vi "Load DXF 2.vi"(7 "DXF Options":T1={"Pen Up Z"=20.0, "Pen Down Z"=-50.0, "Speed"=1500.0, "Z Move Speed"=300.0}, 8 "error in (no error)":errorcluster, 9 "Trigger (SEQEND)":string="SEQEND", 11 "String in":string) -> (0 "error out":errorcluster, 1 "String Array":string[](array[string]), 3 "Command Array":T2[](array[typedef]))   [LabVIEW 2014]
uses:
  GCode Parser/GCode Command Cluster.ctl
panel:
  out "Numeric":i32
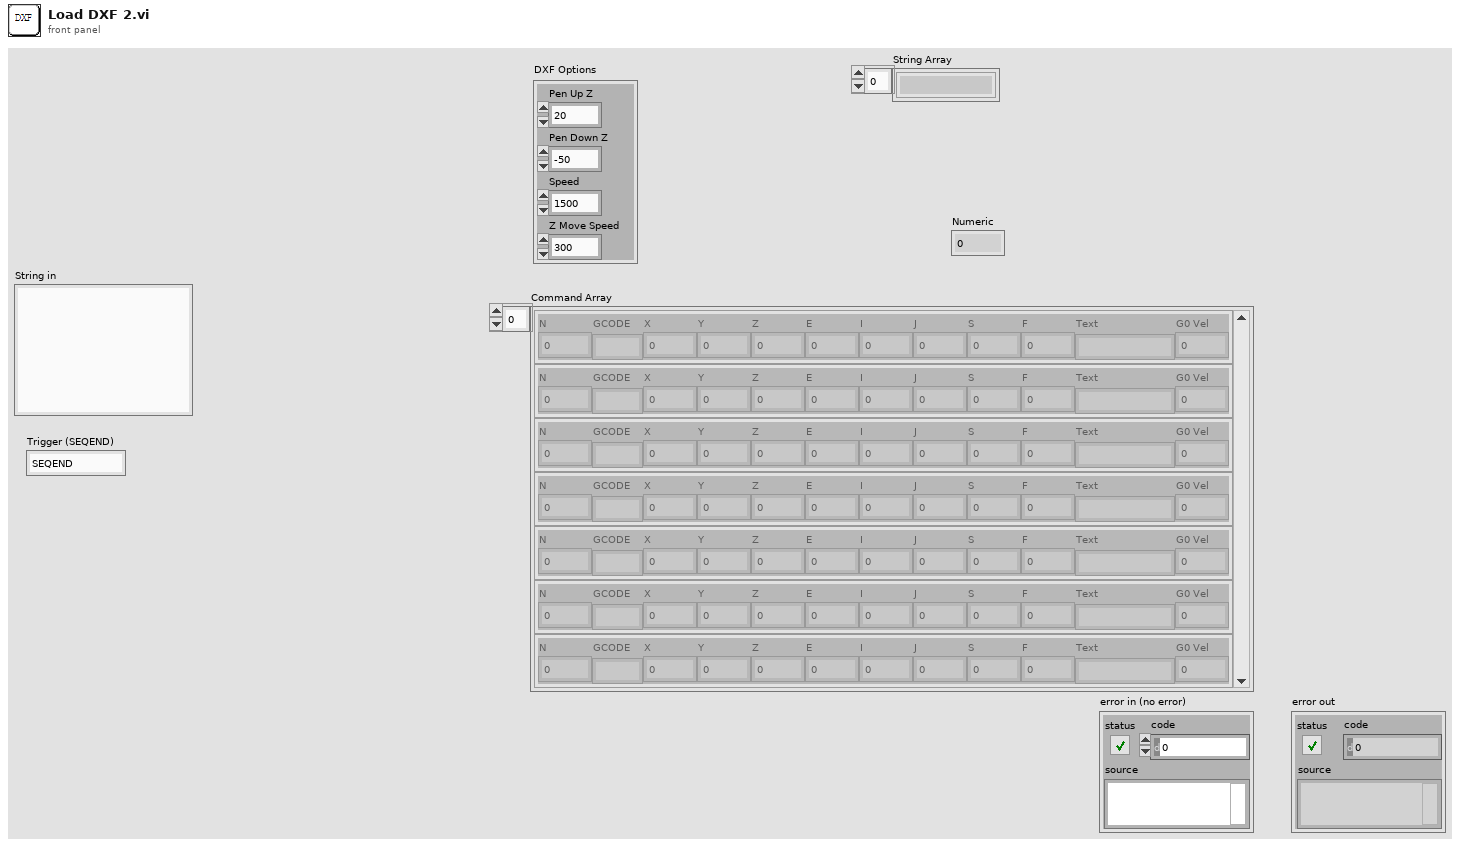
[diagram p1: front panel]
types:
  T1 = cluster{"Pen Up Z":dbl, "Pen Down Z":dbl, "Speed":dbl, "Z Move Speed":dbl}
  T2 = typedef "GCode Command Cluster.ctl" = cluster{"N":dbl, "GCODE":string, "X":dbl, "Y":dbl, "Z":dbl, "E":dbl, "I":dbl, "J":dbl, "S":dbl, "F":dbl, "Text":string, "G0 Vel":dbl}
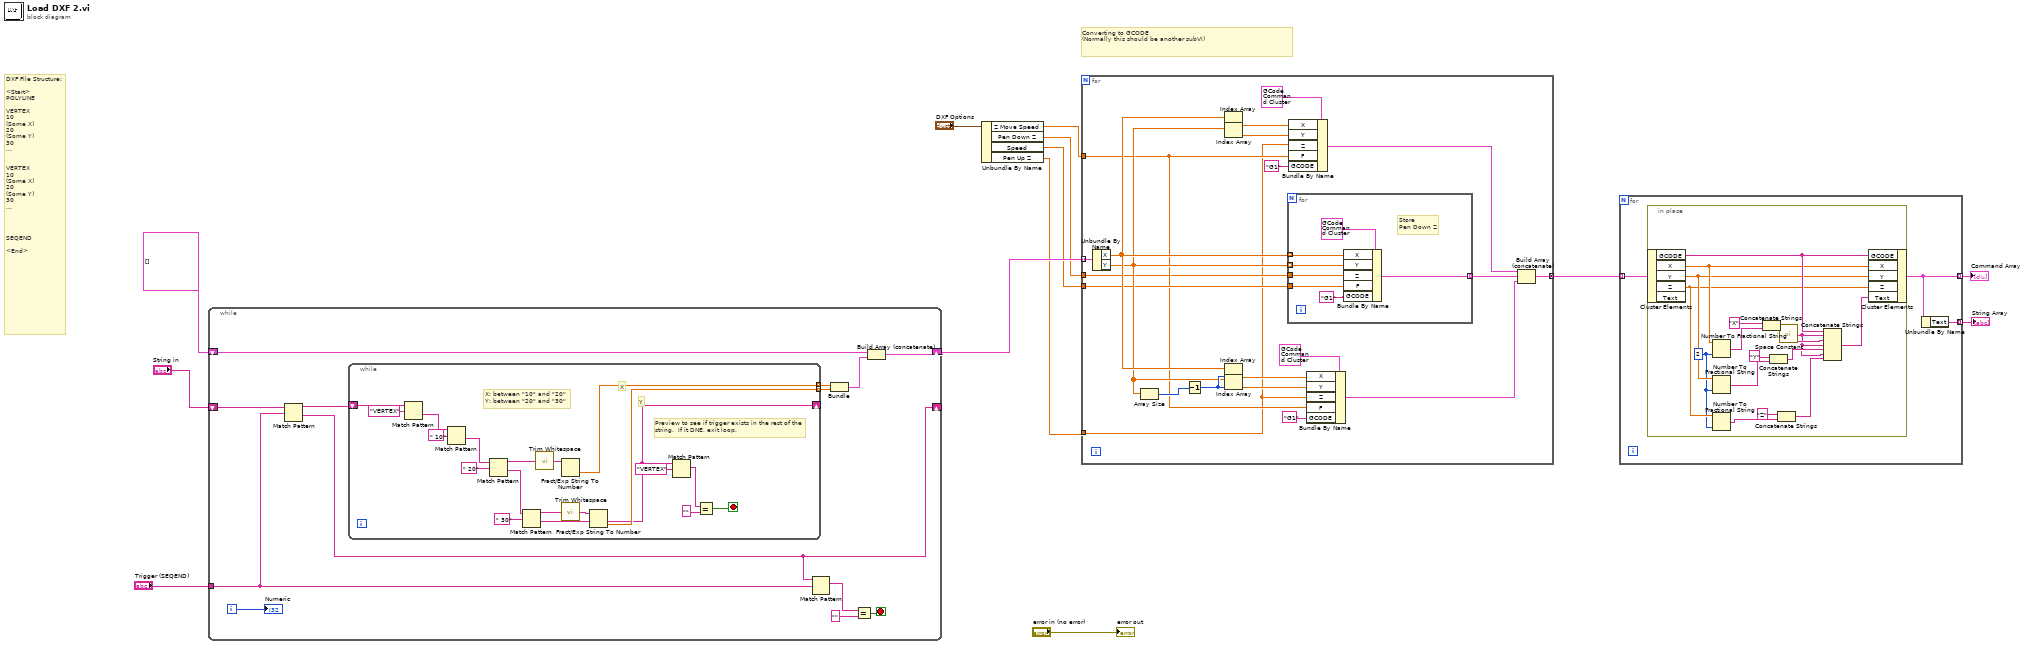
[diagram p0: block diagram]
diagram:
  # "Converting to GCODE\n(Normally this should be another subVI)"
  # "DXF File Structure:\n\n<Start>\nPOLYLINE\n\nVERTEX\n10\n(Some X)\n20\n(Some Y)\n30\n...\n\n\nVERTEX\n10\n(Some X)\n20\n(Some Y)\n30\n...\n\n\n\n\nSEQEND\n\n<End>"
  n1 = while {
    shift-right: [w17] -> _
    shift-left: "String in" -> [w26]
    shift-right: [w14] -> w11
    shift-left: cluster{"X":dbl[], "Y":dbl[]}[] [] -> [w20]
    tunnel: "Trigger (SEQEND)" -> [w15]
    i -> [w19]
    stop <- w24 stop-if-true
    n2 = Match Pattern(string=w26, regular expression=w15) -> (before substring=w18:string, after substring=w17:string)  [unwired: 1 in, 2 out]
    n3 = while {
      shift-right: [w30] -> _
      shift-left: w18 -> [w34]
      tunnel: [w33] -> w23 mode=indexing
      tunnel: [w32] -> w22 mode=indexing
      stop <- w27 stop-if-true
      # "Y"
      # "X"
      # "X: between \"10\" and \"20\" \nY: between \"20\" and \"30\""
      # "Preview to see if trigger exists in the rest of the\nstring.  If it DNE, exit loop."
      n4 = Match Pattern(string=w34, regular expression="VERTEX") -> (after substring=w36:string)  [unwired: 1 in, 3 out]
      n5 = Match Pattern(string=w36, regular expression=" 10") -> (after substring=w35:string)  [unwired: 1 in, 3 out]
      n6 = Match Pattern(string=w35, regular expression=" 20") -> (before substring=w41:string, after substring=w42:string)  [unwired: 1 in, 2 out]
      n7 = Match Pattern(string=w42, regular expression=" 30") -> (before substring=w40:string, after substring=w30:string)  [unwired: 1 in, 2 out]
      n8 = call <vilib>:"Trim Whitespace.vi"("string"=w41) -> ("trimmed string"=w39:string)  [unwired: 1 in]
      n9 = Fract/Exp String To Number(string=w39) -> (number=w33:dbl)  [unwired: 3 in, 1 out]
      n10 = call <vilib>:"Trim Whitespace.vi"("string"=w40) -> ("trimmed string"=w38:string)  [unwired: 1 in]
      n11 = Fract/Exp String To Number(string=w38) -> (number=w32:dbl)  [unwired: 3 in, 1 out]
      n12 = Match Pattern(string=w30, regular expression="VERTEX") -> (match substring=w28:string)  [unwired: 1 in, 3 out]
      n13 = Equal?(x=w28, y="") -> (x = y?=w27:bool)
    }
    n14 = Match Pattern(string=w17, regular expression=w15) -> (match substring=w16:string)  [unwired: 1 in, 3 out]
    n15 = Bundle(w23, w22) -> (w21:cluster{dbl[], dbl[]})  [unwired: 1 in]
    n16 = Equal?(x=w16, y="") -> (x = y?=w24:bool)
    n17 = Build Array (concatenate)(w20, w21) -> (w14:cluster{"X":dbl[], "Y":dbl[]}[])
    "Numeric" <- w19
  }
  n18 = Unbundle By Name("DXF Options") -> ("Z Move Speed"=w8:dbl, "Pen Down Z"=w7:dbl, "Speed"=w6:dbl, "Pen Up Z"=w5:dbl)
  n19 = for {
    tunnel: w11 -> [w66] mode=indexing
    tunnel: [w50] -> w3 mode=concatenating
    tunnel: w6 -> [w49]
    tunnel: w8 -> [w48]
    tunnel: w7 -> [w47]
    tunnel: w5 -> [w46]
    n20 = Unbundle By Name(w66) -> ("X"=w55:dbl[], "Y"=w54:dbl[])
    n21 = Array Size(array=w54) -> (size(s)=w57:i32)
    n22 = Decrement(x=w57) -> (x-1=w56:i32)
    n23 = Index Array(array=w55) -> (element=w65:dbl)  [unwired: 1 in]
    n24 = Index Array(array=w54) -> (element=w64:dbl)  [unwired: 1 in]
    n25 = Index Array(array=w55, index=w56) -> (element=w53:dbl)
    n26 = Index Array(array=w54, index=w56) -> (element=w52:dbl)
    n27 = for {
      tunnel: w55 -> [w73] mode=indexing
      tunnel: w54 -> [w72] mode=indexing
      tunnel: [w71] -> w62 mode=indexing
      tunnel: w49 -> [w68]
      tunnel: w47 -> [w67]
      # "Store\nPen Down Z"
      n28 = Bundle By Name(cluster=T2 {"N"=0.0, "GCODE"="", "X"=0.0, "Y"=0.0, "Z"=0.0, "E"=0.0, "I"=0.0, "J"=0.0, "S"=0.0, "F"=0.0, "Text"="", "G0 Vel"=0.0} ("Cluster 2"), "X"=w73, "Y"=w72, "Z"=w67, "F"=w68, "GCODE"="G1") -> (w71:T2)
    }
    n29 = Bundle By Name(cluster=T2 {"N"=0.0, "GCODE"="", "X"=0.0, "Y"=0.0, "Z"=0.0, "E"=0.0, "I"=0.0, "J"=0.0, "S"=0.0, "F"=0.0, "Text"="", "G0 Vel"=0.0} ("Cluster 2"), "X"=w65, "Y"=w64, "Z"=w46, "F"=w48, "GCODE"="G1") -> (w60:T2)
    n30 = Bundle By Name(cluster=T2 {"N"=0.0, "GCODE"="", "X"=0.0, "Y"=0.0, "Z"=0.0, "E"=0.0, "I"=0.0, "J"=0.0, "S"=0.0, "F"=0.0, "Text"="", "G0 Vel"=0.0} ("Cluster 2"), "X"=w53, "Y"=w52, "Z"=w46, "F"=w48, "GCODE"="G1") -> (w51:T2)
    n31 = Build Array (concatenate)(w60, w62, w51) -> (w50:T2[])
  }
  n32 = for {
    tunnel: w3 -> [w76] mode=indexing
    tunnel: [w75] -> w2 mode=indexing
    tunnel: [w74] -> w1 mode=indexing
    n33 = in-place {
      w77 = i16 2 ("precision (6)")
      n34 = in-place-cluster #1(w76) -> ("GCODE"=w81:string, "X"=w80:dbl, "Y"=w79:dbl, "Z"=w78:dbl)  [unwired: 1 out]
      n35 = Number To Fractional String(number=w80, precision (6)=w77) -> (F-format string=w91:string)  [unwired: 2 in]
      n36 = Number To Fractional String(number=w79, precision (6)=w77) -> (F-format string=w90:string)  [unwired: 2 in]
      n37 = Number To Fractional String(number=w78, precision (6)=w77) -> (F-format string=w89:string)  [unwired: 2 in]
      n38 = Concatenate Strings("X", w91) -> (w86:string)
      n39 = Concatenate Strings("Y" ("string"), w90) -> (w85:string)
      n40 = Concatenate Strings("Z" ("string"), w89) -> (w83:string)
      n41 = call <vilib>:"Space Constant.vi"() -> ("String"=w84:string)
      n42 = Concatenate Strings(w81, w84, w86, w84, w85, w84, w83) -> (w82:string)
      n43 = in-place-cluster #1("GCODE"=w81, "X"=w80, "Y"=w79, "Z"=w78, "Text"=w82) -> (w75:T2)
    }
    n44 = Unbundle By Name(w75) -> ("Text"=w74:string)
  }
  "Command Array" <- w2
  "String Array" <- w1
  "error out" <- "error in (no error)"
